vi "loadSomeRFPDataFiles.vi"(4 "Length":i32, 6 "Index":i32, 7 "File Types to Read":T1, 9 "File Index":i32, 10 "Files":path[](array[path]), 11 "Template":path) -> (1 "rowNumbers":i32[][](array[numeric]), 2 "Channel Values Out":string[][](array[string]), 3 "filetypes":string[](array[string]), 5 "Ch names Out":string[](array[string]))   [LabVIEW 2022 SP3]
uses:
  Anemometry/Anemometry Sub Vis/Data_plotting_vis/Data_File_Type.ctl
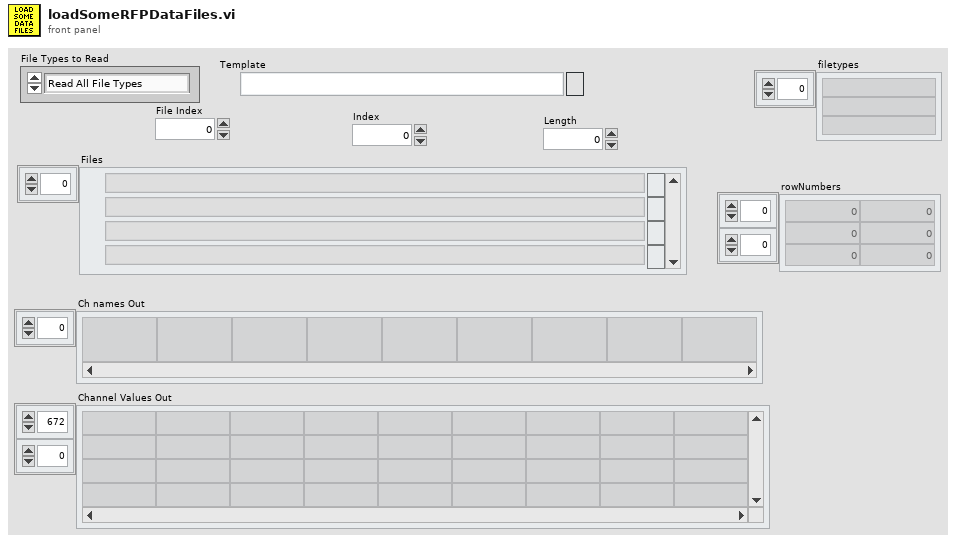
[diagram p1: front panel]
types:
  T1 = typedef "Data_File_Type.ctl" = enum16{"Read All File Types", "Results Files Only", "Raw Data Files Only", "Calibration Files Only", "Gas Desk Files Only", "Old Results Files Only", "Tabulated Data Files Only"}
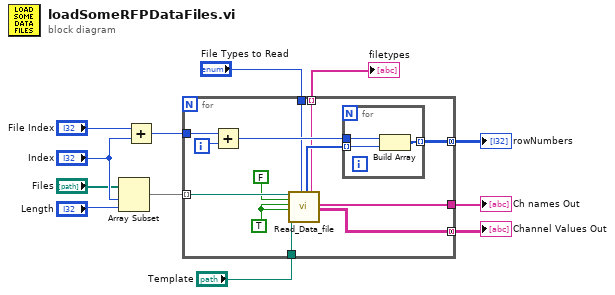
[diagram p0: block diagram]
diagram:
  n1 = Array Subset(array="Files", index="Index", length="Length") -> (w3:path[])
  n2 = Add(x="File Index", y="Index") -> (x+y=w5:i32)
  n3 = for {
    tunnel: "Template" -> [w25]
    tunnel: w3 -> [w24] mode=indexing
    tunnel: [w22] -> w7 mode=concatenating
    tunnel: [w21] -> w4
    tunnel: w5 -> [w19]
    tunnel: [w16] -> w9 mode=concatenating
    tunnel: [w15] -> w8 mode=indexing
    tunnel: "File Types to Read" -> [w14]
    i -> [w20]
    w13 = TRUE ("Delete First Rows?")
    n4 = Add(x=w19, y=w20) -> (x+y=w18:i32)
    n5 = call "Read_Data_file.vi"("Results file"=w24, "Read Channel Names only"=FALSE, "Delete First Rows?"=w13, "Add Extra Channels?"=w13, "Template File"=w25, "Desired File Types"=w14) -> ("Row numbers"=w17:i32[], "Filetype"=w15:string, "Ch names Out"=w21:string[], "Channel Values Out"=w22:string[][])  [unwired: 1 in, 9 out]
    n6 = for {
      tunnel: w18 -> [w28]
      tunnel: [w27] -> w16 mode=indexing
      tunnel: w17 -> [w26] mode=indexing
      n7 = Build Array(w28, w26) -> (w27:i32[])
    }
  }
  "rowNumbers" <- w9
  "filetypes" <- w8
  "Channel Values Out" <- w7
  "Ch names Out" <- w4
